vi "Host Approach Retraction2(1).vi"() -> ()   [LabVIEW 2012]
uses:
  <vilib>/FPGAPlugInAG/PCI-7831R/niLvFpga_Open_PCI-7831R.vi
  <vilib>/rvi/interface/common/dynamic/niFpgaDynamicAddResources.vi
  <vilib>/Utility/error.llb/Error Cluster From Error Code.vi
  <vilib>/rvi/errors/niLvFpgaAdjustHostInterfaceError.vi
  <vilib>/FPGAPlugInAG/Dynamic/niLvFpga_Close_Dynamic.vi
  <vilib>/FPGAPlugInAG/Dynamic/niLvFpga_Run_Dynamic.vi
  <vilib>/rvi/interface/nirviOpenFPGA/nirviOpenFPGA.xnode
  SB130-XPS/Documents/FPGA-project-apporach-retraction/FPGA Bitfiles/Apporach-Retract_FPGATarget2_FPGATargetApproa_0M-AxT4gclo.lvbitx
  FPGA Target Approach Retraction2(2).vi
  <vilib>/rvi/interface/nirviReadWriteControl/nirviReadWriteControl.xnode
  <vilib>/rvi/interface/nirviCloseFPGA/nirviCloseFPGA.xnode
  <vilib>/rvi/interface/nirviMethod/nirviMethod.xnode
  <vilib>/rvi/interface/Simulation/niFpgaSimulationCallBeginRW.vi
  <vilib>/rvi/errors/niLvFpgaMergeErrorWithErrorCode.vi
  NiFpgaLv.dll
  <vilib>/FPGAPlugInAG/Dynamic/niLvFpga_StartFifo_Dynamic.vi
  <vilib>/FPGAPlugInAG/Dynamic/niLvFpga_StopFifo_Dynamic.vi
  <vilib>/FPGAPlugInAG/Dynamic/niLvFpga_ReadFifo_Dynamic.vi
panel:
  out "CO2":dbl(graph)
  in  "Bit/nm converter":fxp<+,26,2>
  in  "Fast Approach Speed (nm/s)":i32
  in  "Automated Approach Start":bool
  in  "Data Acquisition Rate (us)":i32
  out "HV/10":i32[](graph)
  out "Tuning Fork Signal":i32[](graph)
  out "Array":i64[](array[numeric])
  in  "Number of Elements":u16
  out "Counter Indicator":i32(graph)
  out "Z Indicator":dbl(graph)
  out "FPGA Output Voltage":dbl(graph)
  in  "MCL Counter":i64
  in  "MCL Divisions":i32
  out "MCL Range Indicator":bool
  out "Host Counter Indicator":i64
  out "Digital Steps per Region":i32
  out "Host Counter Output":i32
  in  "Z Position MCL Fine":i32
  out "Host Z Position Indicator":i32
  out "Z Position Range Indicator":bool
  out "Z Fine Steps per Region":dbl
  out "Host Z Output":fxp<+/-,40,30>
  in  "Manual Approach Start":bool
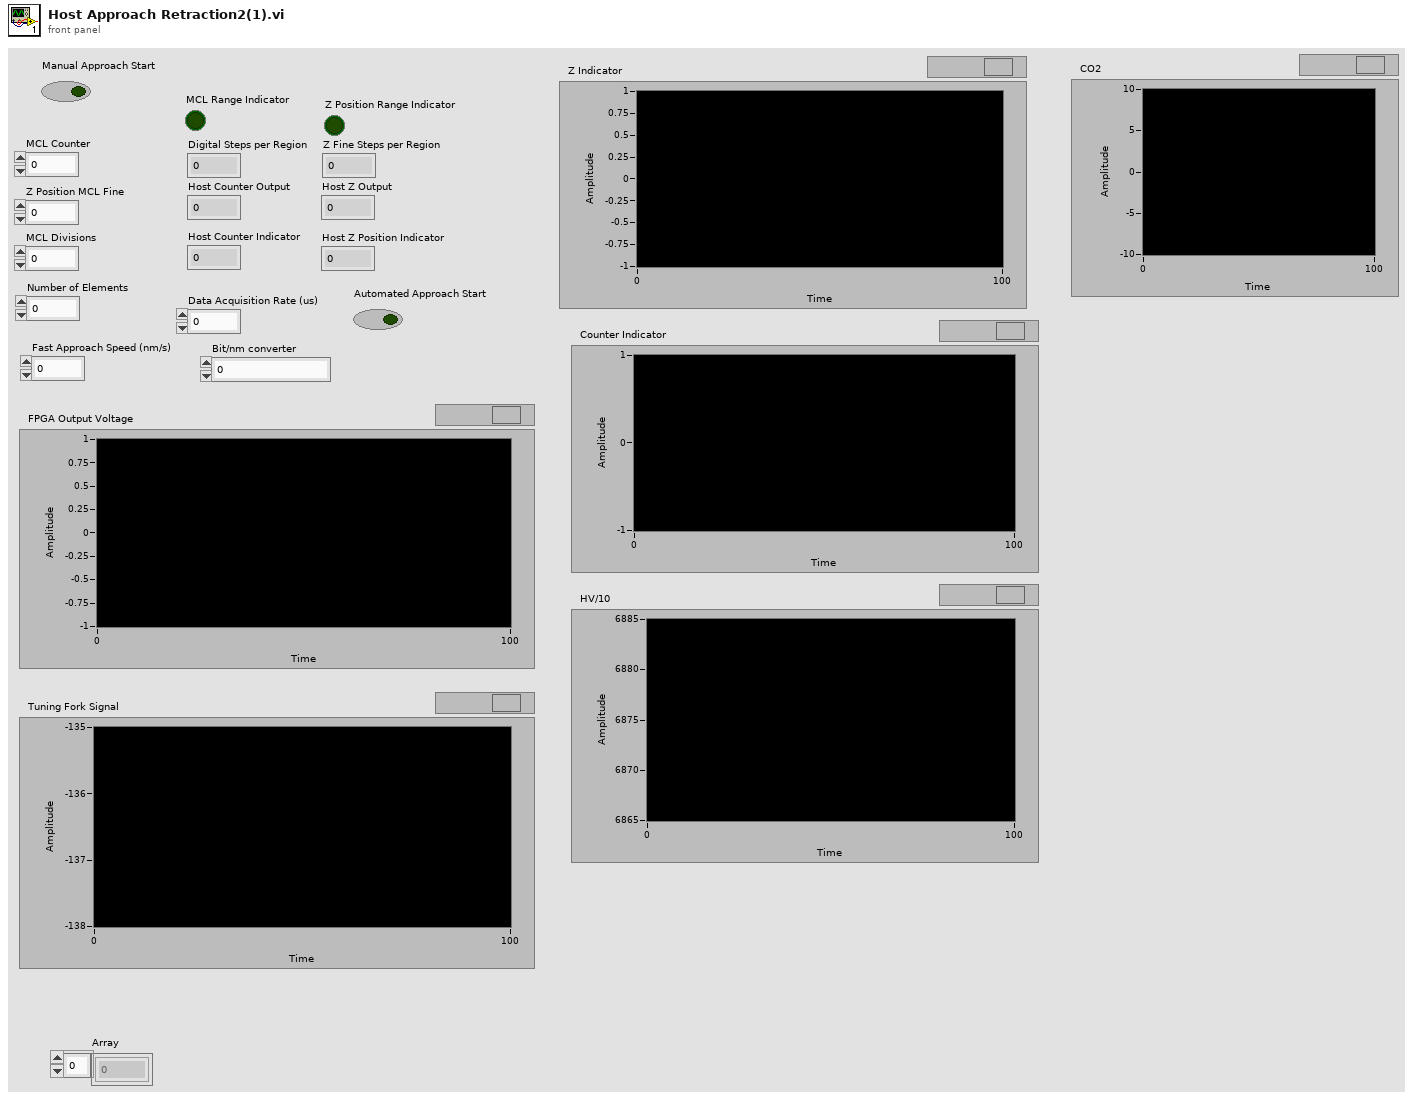
[diagram p1: front panel]
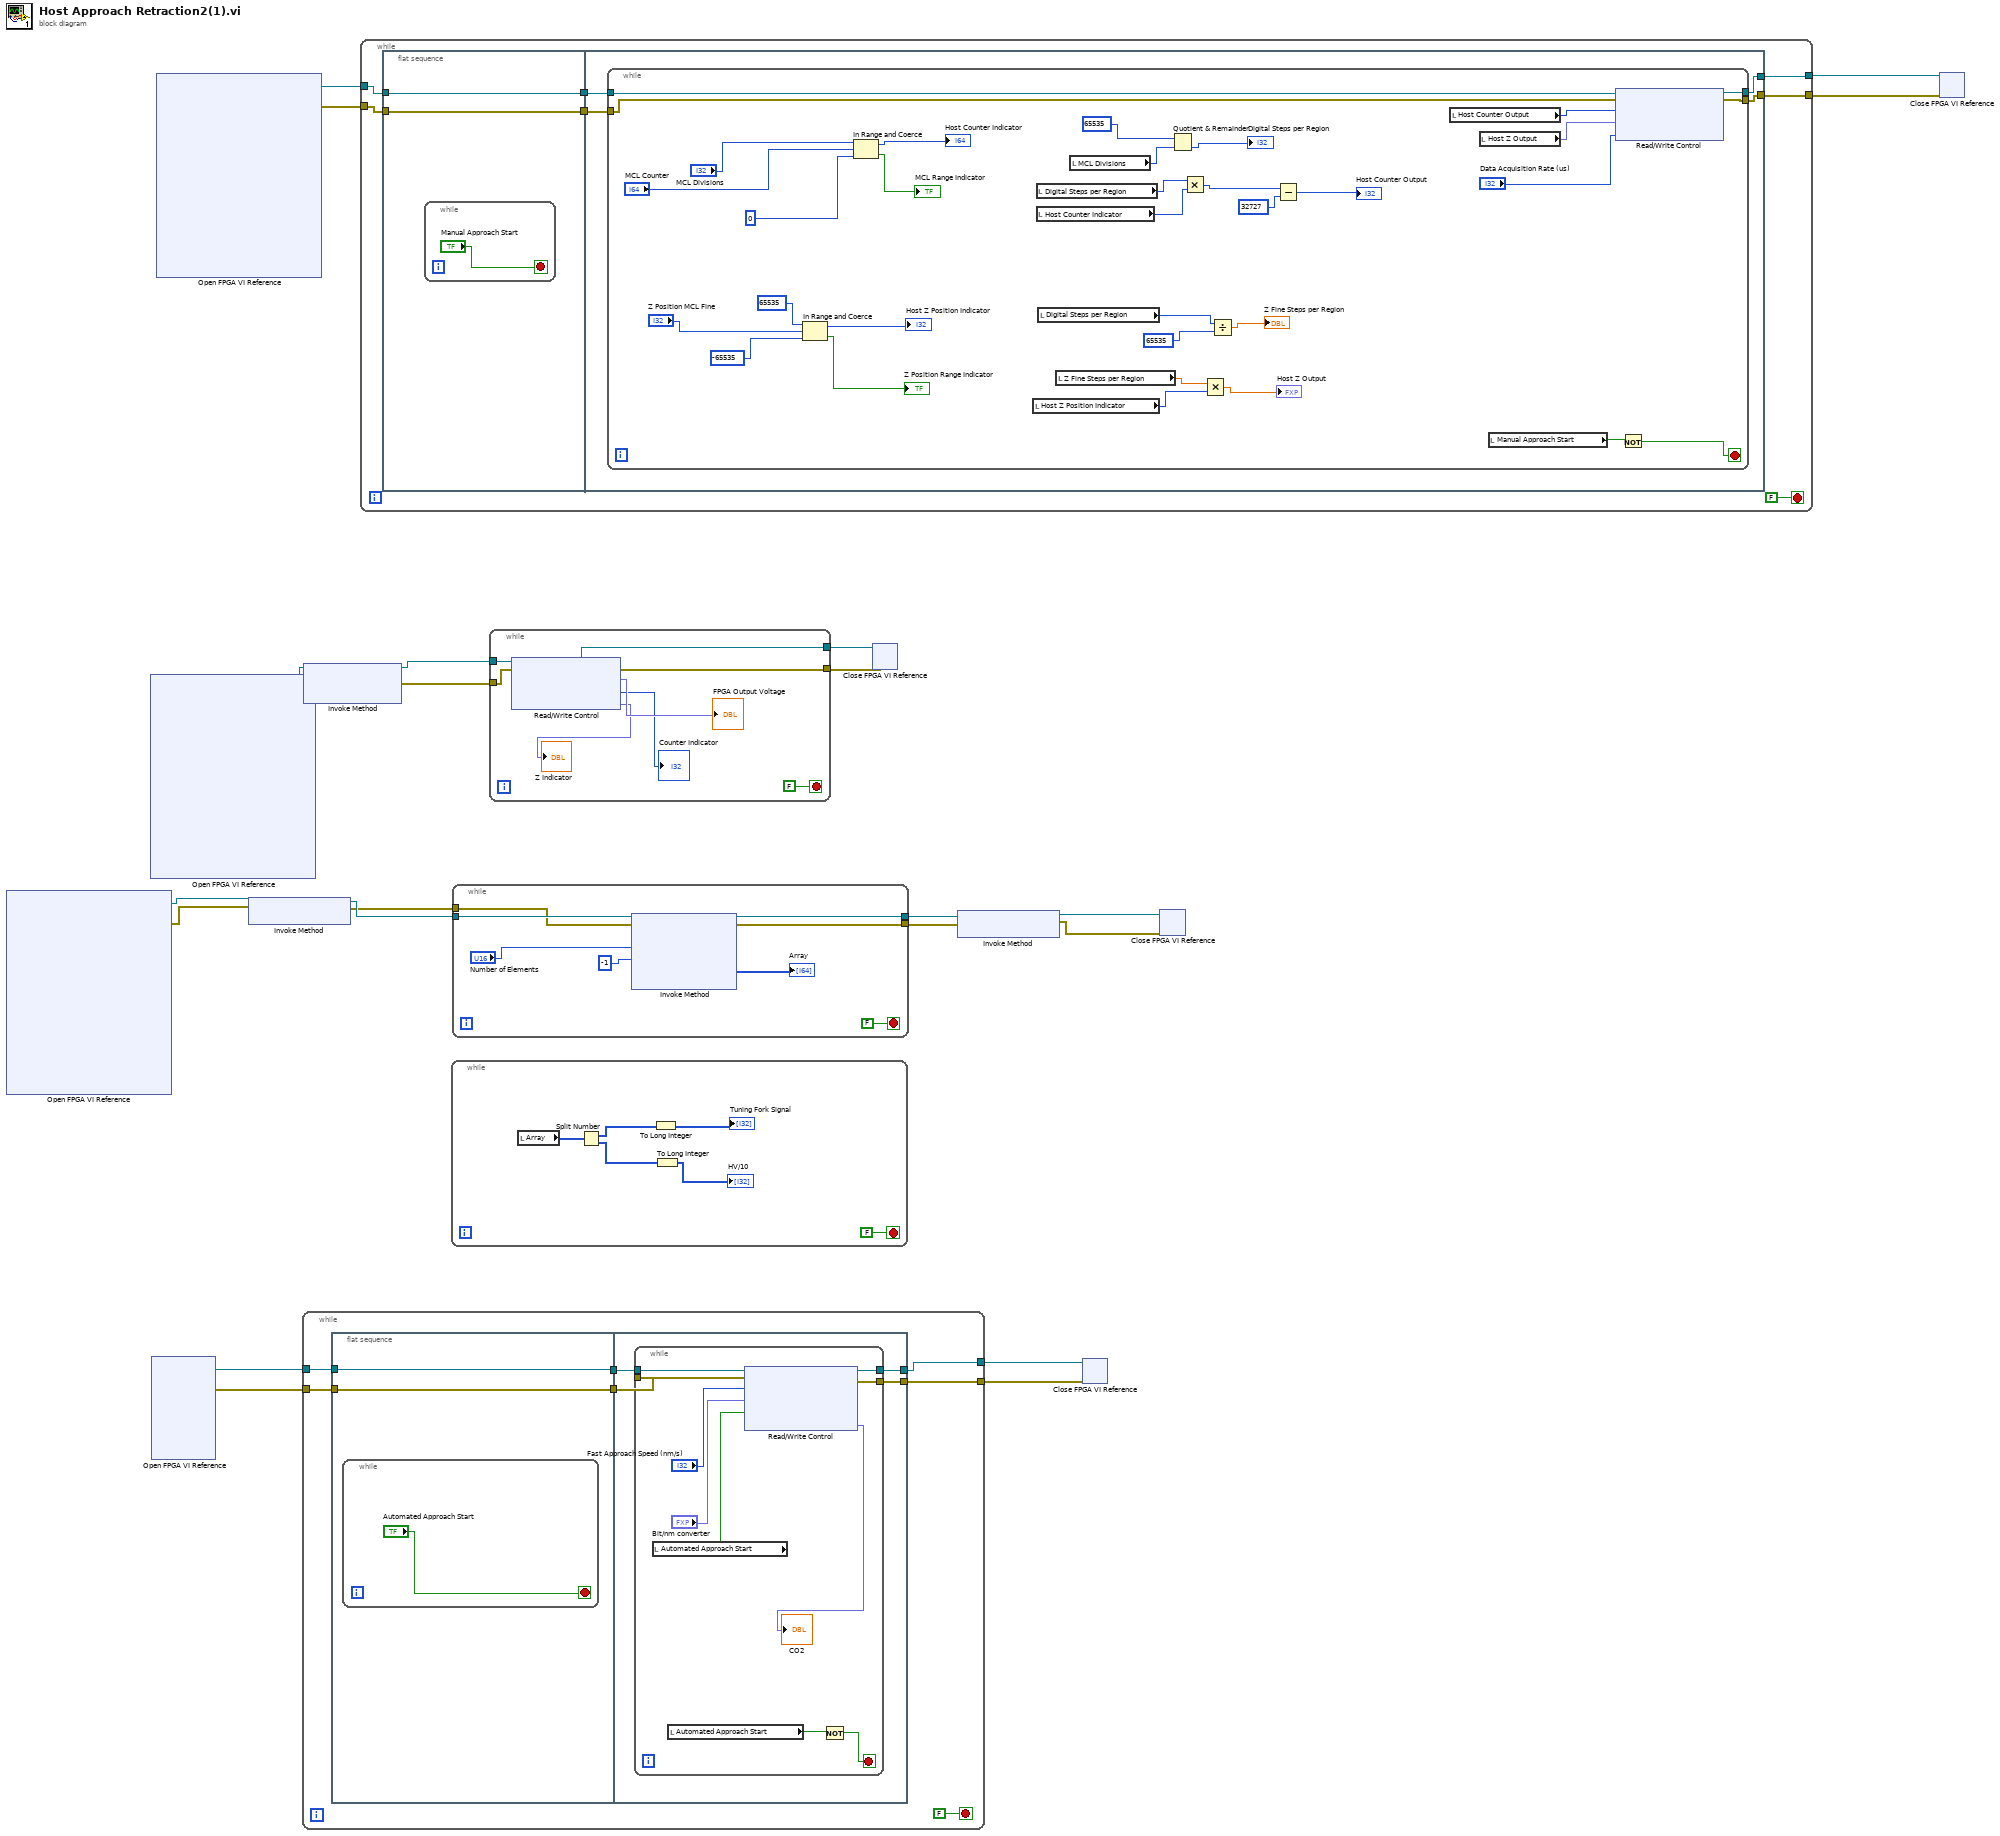
[diagram p0: block diagram]
diagram:
  n1 = xnode "Open FPGA VI Reference"() -> ("FPGA VI Reference Out"=w12:refnum<k20>, "error out"=w11:errorcluster)  [unwired: 2 in]
  n2 = xnode "Open FPGA VI Reference"() -> ("FPGA VI Reference Out"=w14:refnum<k20>, "error out"=w13:errorcluster)  [unwired: 2 in]
  n3 = xnode "Open FPGA VI Reference"() -> ("FPGA VI Reference Out"=w4:refnum<k20>, "error out"=w3:errorcluster)  [unwired: 2 in]
  n4 = xnode "Open FPGA VI Reference"() -> ("FPGA VI Reference Out"=w20:refnum<k20>, "error out"=w19:errorcluster)  [unwired: 2 in]
  n5 = xnode "Invoke Method"("FPGA VI Reference In"=w12, "error in"=w11) -> ("FPGA VI Reference Out"=w10:refnum<k20>, "error out"=w9:errorcluster)
  n6 = while {
    tunnel: w4 -> [w28]
    tunnel: w3 -> [w27]
    tunnel: [w24] -> w2
    tunnel: [w23] -> w1
    stop <- FALSE stop-if-true
    n7 = flat-sequence {
      tunnel: w28 -> [w31]
      tunnel: w27 -> [w30]
      tunnel: [w31] -> w26
      tunnel: [w30] -> w25
      tunnel: w26 -> [w36]
      tunnel: w25 -> [w35]
      tunnel: [w34] -> w24
      tunnel: [w33] -> w23
      frame #0 {
        n8 = while {
          stop <- "Automated Approach Start" stop-if-true
        }
      }
      frame #1 {
        n9 = while {
          tunnel: w36 -> [w46]
          tunnel: w35 -> [w45]
          tunnel: [w44] -> w34
          tunnel: [w43] -> w33
          stop <- w41 stop-if-true
          n10 = local read "Automated Approach Start"() -> (w39:bool)
          n11 = local read "Automated Approach Start"() -> (w42:bool)
          n12 = xnode "Read/Write Control"("FPGA VI Reference In"=w46, "error in"=w45, "Fast Approach Speed"="Fast Approach Speed (nm/s)", "Bit/nm converter"="Bit/nm converter", "Automated FPGA Start"=w39) -> ("FPGA VI Reference Out"=w44:refnum<k20>, "error out"=w43:errorcluster, "Counter Output 2"=→"CO2":fxp<+/-,16,16>)
          n13 = Not(x=w42) -> (.not. x?=w41:bool)
        }
      }
    }
  }
  n14 = xnode "Invoke Method"("FPGA VI Reference In"=w14, "error in"=w13) -> ("FPGA VI Reference Out"=w16:refnum<k20>, "error out"=w15:errorcluster)  [unwired: 1 in]
  n15 = while {
    tunnel: [w52] -> w22
    tunnel: [w51] -> w21
    tunnel: w20 -> [w49]
    tunnel: w19 -> [w47]
    stop <- FALSE stop-if-true
    n16 = flat-sequence {
      tunnel: [w55] -> w50
      tunnel: w49 -> [w55]
      tunnel: [w54] -> w48
      tunnel: w47 -> [w54]
      tunnel: [w58] -> w52
      tunnel: [w57] -> w51
      tunnel: w50 -> [w60]
      tunnel: w48 -> [w59]
      frame #0 {
        n17 = while {
          stop <- "Manual Approach Start" stop-if-true
        }
      }
      frame #1 {
        n18 = while {
          tunnel: w60 -> [w93]
          tunnel: w59 -> [w92]
          tunnel: [w91] -> w58
          tunnel: [w90] -> w57
          stop <- w88 stop-if-true
          n19 = In Range and Coerce(upper limit=65535, x="Z Position MCL Fine", lower limit=-65535) -> (coerced(x)=→"Host Z Position Indicator":i32, In Range?=→"Z Position Range Indicator":bool)
          n20 = In Range and Coerce(upper limit="MCL Divisions", x="MCL Counter", lower limit=0) -> (coerced(x)=→"Host Counter Indicator":i64, In Range?=→"MCL Range Indicator":bool)
          n21 = local read "Host Z Position Indicator"() -> (w64:i32)
          n22 = local read "Digital Steps per Region"() -> (w77:i32)
          n23 = local read "Host Counter Indicator"() -> (w76:i64)
          n24 = local read "Digital Steps per Region"() -> (w68:i32)
          n25 = local read "Z Fine Steps per Region"() -> (w65:dbl)
          n26 = local read "MCL Divisions"() -> (w81:i32)
          n27 = Quotient & Remainder(x=65535, y=w81) -> (floor(x/y)=→"Digital Steps per Region":i32)  [unwired: 1 out]
          n28 = Multiply(x=w77, y=w76) -> (x*y=w78:i64)
          n29 = Multiply(x=w65, y=w64) -> (x*y=→"Host Z Output":dbl)
          n30 = Divide(x=w68, y=65535) -> (x/y=→"Z Fine Steps per Region":dbl)
          n31 = Subtract(x=w78, y=32727) -> (x-y=→"Host Counter Output":i64)
          n32 = local read "Host Counter Output"() -> (w74:i32)
          n33 = local read "Host Z Output"() -> (w62:fxp<+/-,40,30>)
          n34 = local read "Manual Approach Start"() -> (w89:bool)
          n35 = xnode "Read/Write Control"("FPGA VI Reference In"=w93, "error in"=w92, "Counter Output"=w74, "Z Fine Output"=w62, "Data Acquisition Rate"="Data Acquisition Rate (us)") -> ("FPGA VI Reference Out"=w91:refnum<k20>, "error out"=w90:errorcluster)
          n36 = Not(x=w89) -> (.not. x?=w88:bool)
        }
      }
    }
  }
  n37 = while {
    stop <- FALSE stop-if-true
    n38 = local read "Array"() -> (w99:i64[])
    n39 = Split Number(x=w99) -> (hi(x)=w95:u32[], lo(x)=w97:u32[])
    n40 = To Long Integer(number=w95) -> (32bit integer=→"Tuning Fork Signal":i32[])
    n41 = To Long Integer(number=w97) -> (32bit integer=→"HV/10":i32[])
  }
  n42 = while {
    tunnel: w10 -> [w107]
    tunnel: w9 -> [w106]
    tunnel: [w105] -> w8
    tunnel: [w104] -> w7
    stop <- FALSE stop-if-true
    n43 = xnode "Invoke Method"("FPGA VI Reference In"=w107, "error in"=w106, "Number of Elements"="Number of Elements", "Timeout (ms)"=-1) -> ("FPGA VI Reference Out"=w105:refnum<k20>, "error out"=w104:errorcluster, "Data"=→"Array":i64[])  [unwired: 1 out]
  }
  n44 = while {
    tunnel: w16 -> [w114]
    tunnel: w15 -> [w113]
    tunnel: [w112] -> w18
    tunnel: [w111] -> w17
    stop <- FALSE stop-if-true
    n45 = xnode "Read/Write Control"("FPGA VI Reference In"=w114, "error in"=w113) -> ("FPGA VI Reference Out"=w112:refnum<k20>, "error out"=w111:errorcluster, "FPGA Output Voltage"=→"FPGA Output Voltage":fxp<+/-,64,32>, "Counter Indicator"=→"Counter Indicator":i32, "Z Fine Indicator"=→"Z Indicator":fxp<+/-,40,30>)
  }
  n46 = xnode "Close FPGA VI Reference"("FPGA VI Reference In"=w18, "error in"=w17) -> ()  [unwired: 1 out]
  n47 = xnode "Invoke Method"("FPGA VI Reference In"=w8, "error in"=w7) -> ("FPGA VI Reference Out"=w6:refnum<k20>, "error out"=w5:errorcluster)
  n48 = xnode "Close FPGA VI Reference"("FPGA VI Reference In"=w2, "error in"=w1) -> ()  [unwired: 1 out]
  n49 = xnode "Close FPGA VI Reference"("FPGA VI Reference In"=w6, "error in"=w5) -> ()  [unwired: 1 out]
  n50 = xnode "Close FPGA VI Reference"("FPGA VI Reference In"=w22, "error in"=w21) -> ()  [unwired: 1 out]
